vi "Update from Right.vi"(9 "Col":i32, 10 "Row":i32, 11 "Proto in":refnum<class "Proto.lvclass">) -> (3 "Proto out":refnum<class "Proto.lvclass">)   [LabVIEW 2021, in "Proto.lvclass"]
uses:
  Proto.lvclass
  Proto.lvclass/Proto.ctl
  Direction.ctl
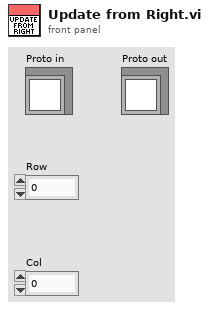
[diagram p1: front panel]
types:
  T1 = typedef "Proto.lvclass/Direction.ctl" = enum16{"Up", "Down", "Right", "Left"}
  T2 = map{cluster{"Row":i32, "Col":i32}, set{cluster{"Heat":i32, "Prev Steps":T1[]}}}
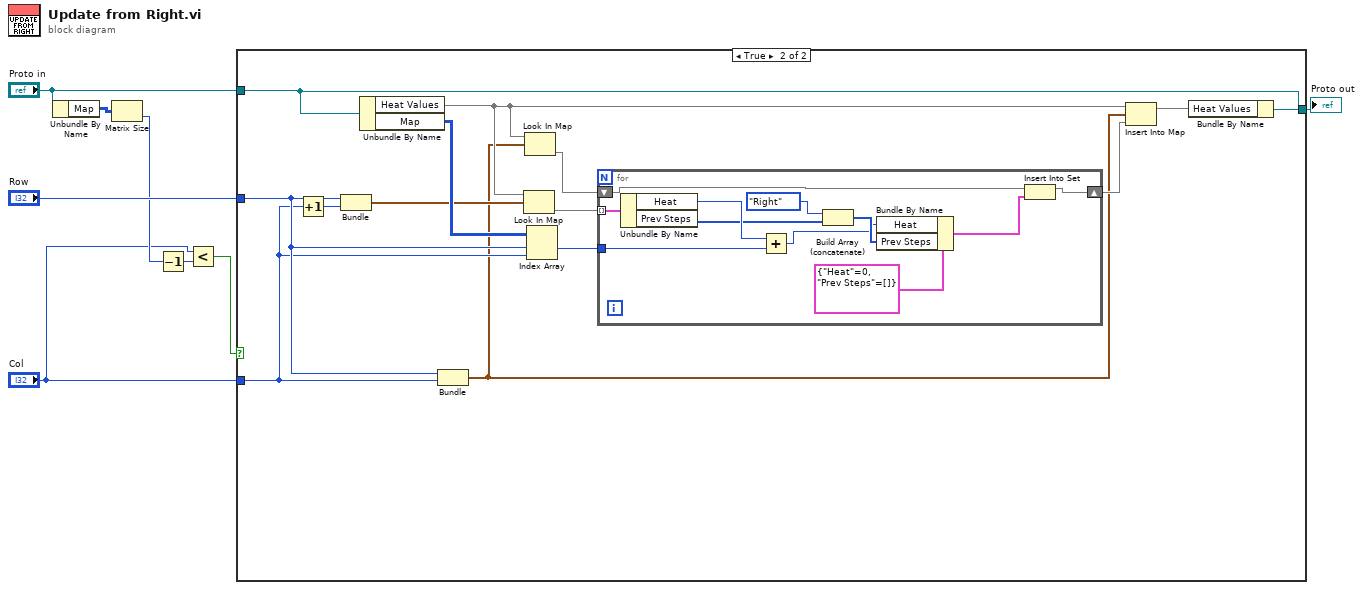
[diagram p0: block diagram]
diagram:
  n1 = Unbundle By Name("Proto in") -> ("Map"=w5:i32[][])
  n2 = Matrix Size(0:w5) -> (2:w4:i32)  [unwired: 1 out]
  n3 = Decrement(x=w4) -> (x-1=w2:i32)
  n4 = Less?(x="Col", y=w2) -> (x < y?=w3:bool)
  n5 = case shown="True" w3 {
    tunnel: [w9 w21] -> w8
    tunnel: "Proto in" -> [w9 w20]
    tunnel: "Row" -> [_ w17]
    tunnel: "Col" -> [_ w16]
    frame False {
    }
    frame True {
      n6 = Increment(x=w16) -> (x+1=w15:i32)
      n7 = Bundle("Row"=w17, w15) -> (w19:cluster{"Row":i32, i32})  [unwired: 1 in]
      n8 = Unbundle By Name(w20) -> ("Heat Values"=w12:T2, "Map"=w23:i32[][])
      n9 = Bundle("Row"=w17, "Col"=w16) -> (w11:cluster{"Row":i32, "Col":i32})  [unwired: 1 in]
      n10 = Look In Map(map=w12, key=w19) -> (value=w14:set{cluster{"Heat":i32, "Prev Steps":T1[]}})  [unwired: 1 in, 1 out]
      n11 = Look In Map(map=w12, key=w11) -> (value=w10:set{cluster{"Heat":i32, "Prev Steps":T1[]}})  [unwired: 1 in, 1 out]
      n12 = Index Array(array=w23, index (row)=w17, index (col)=w16) -> (element=w18:i32)
      n13 = for {
        tunnel: w14 -> [w30] mode=indexing
        tunnel: w18 -> [w33]
        shift-right: [w26] -> w13
        shift-left: w10 -> [w27]
        n14 = Unbundle By Name(w30) -> ("Heat"=w34:i32, "Prev Steps"=w32:T1[])
        n15 = Add(x=w34, y=w33) -> (x+y=w28:i32)
        n16 = Build Array (concatenate)(Direction."Right" ("Dir"), w32) -> (w29:T1[])
        n17 = Bundle By Name(cluster=cluster{"Heat":i32, "Prev Steps":T1[]} {"Heat"=0, "Prev Steps"=[]} ("element"), "Heat"=w28, "Prev Steps"=w29) -> (w25:cluster{"Heat":i32, "Prev Steps":T1[]})
        n18 = Insert Into Set(10:w25, 11:w27) -> (3:w26:set{cluster{"Heat":i32, "Prev Steps":T1[]}})  [unwired: 1 out]
      }
      n19 = Insert Into Map(map in=w12, key=w11, value=w13) -> (map out=w22:T2)  [unwired: 2 out]
      n20 = Bundle By Name(cluster=w20, "Heat Values"=w22) -> (w21:refnum<class "Proto.lvclass">)
    }
  }
  "Proto out" <- w8
